vi "act.vi"(4 "V":i8, 5 "Ein":i8, 6 "Yin":i8, 7 "Xin":i8, 8 "Input Array":i8[][](array[numeric])) -> (0 "Eout":i8, 1 "Yout":i8, 2 "Xout":i8, 3 "Output Array":i8[][](array[numeric]))   [LabVIEW 2012]
doc: "This VI moves the robot based on a given heading* and updates its attributes, including energy, accondingly.\n\nHeadings:\n6 7 8\n5 0 1\n4 3 2"
panel:
  # "V Code\n  6 7 8\n  5 0 1\n  4 3 2"
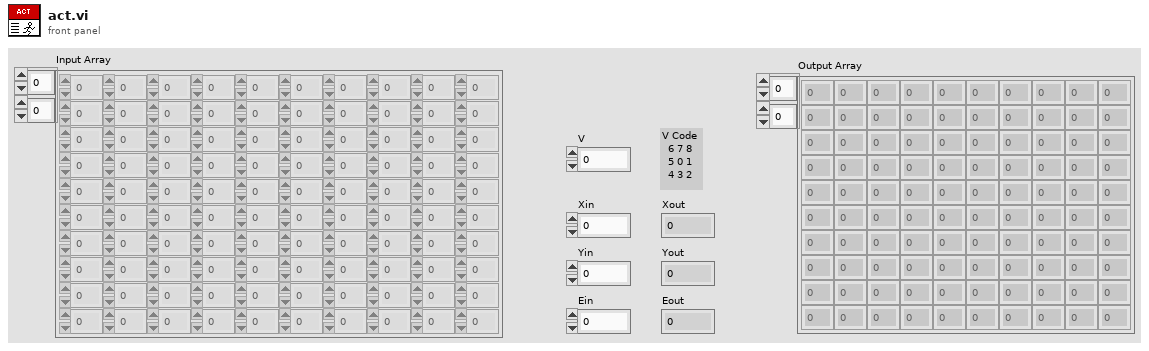
[diagram p1: front panel]
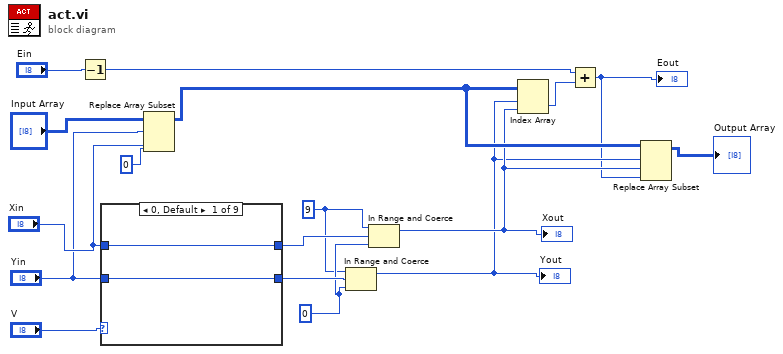
[diagram p0: block diagram]
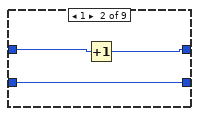
[diagram p2: hidden frame]
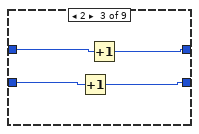
[diagram p3: hidden frame]
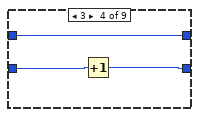
[diagram p4: hidden frame]
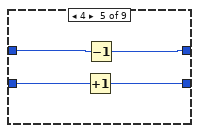
[diagram p5: hidden frame]
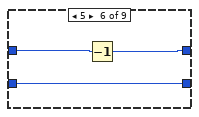
[diagram p6: hidden frame]
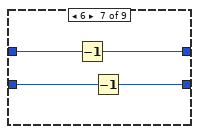
[diagram p7: hidden frame]
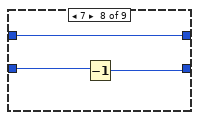
[diagram p8: hidden frame]
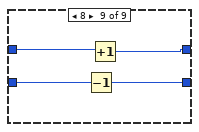
[diagram p9: hidden frame]
diagram:
  w8 = i8 0
  w7 = i8 9
  n1 = Decrement(x="Ein") -> (x-1=w16:i8)
  n2 = case shown="0, Default" "V" {
    tunnel: "Xin" -> [w19 w21 w26 w29 w31 w35 w37 w43 w45]
    tunnel: "Yin" -> [w18 w22 w23 w27 w33 w36 w40 w42 w47]
    tunnel: [w19 w20 w25 w29 w30 w34 w38 w43 w44] -> w9
    tunnel: [w18 w22 w24 w28 w32 w36 w39 w41 w46] -> w10
    frame 0, Default {
    }
    frame 1 {
      n3 = Increment(x=w21) -> (x+1=w20:i8)
    }
    frame 2 {
      n4 = Increment(x=w23) -> (x+1=w24:i8)
      n5 = Increment(x=w26) -> (x+1=w25:i8)
    }
    frame 3 {
      n6 = Increment(x=w27) -> (x+1=w28:i8)
    }
    frame 4 {
      n7 = Increment(x=w33) -> (x+1=w32:i8)
      n8 = Decrement(x=w31) -> (x-1=w30:i8)
    }
    frame 5 {
      n9 = Decrement(x=w35) -> (x-1=w34:i8)
    }
    frame 6 {
      n10 = Decrement(x=w37) -> (x-1=w38:i8)
      n11 = Decrement(x=w40) -> (x-1=w39:i8)
    }
    frame 7 {
      n12 = Decrement(x=w42) -> (x-1=w41:i8)
    }
    frame 8 {
      n13 = Decrement(x=w47) -> (x-1=w46:i8)
      n14 = Increment(x=w45) -> (x+1=w44:i8)
    }
  }
  n15 = Replace Array Subset(array="Input Array", new element=i8 0, index (row)="Yin", index (col)="Xin") -> (w12:i8[][])
  n16 = In Range and Coerce(upper limit=w7, x=w10, lower limit=w8) -> (coerced(x)=w5:i8)  [unwired: 1 out]
  "Yout" <- w5
  n17 = In Range and Coerce(upper limit=w7, x=w9, lower limit=w8) -> (coerced(x)=w6:i8)  [unwired: 1 out]
  "Xout" <- w6
  n18 = Index Array(array=w12, index (row)=w5, index (col)=w6) -> (element=w14:i8)
  n19 = Add(x=w16, y=w14) -> (x+y=w4:i8)
  "Eout" <- w4
  n20 = Replace Array Subset(array=w12, new element=w4, index (row)=w5, index (col)=w6) -> (→"Output Array":i8[][])
